vi "LCW_Flow_Mon_Main.vi"() -> ()   [LabVIEW 2019]
uses:
  <vilib>/MakerHub/LINX/LMH-LINX.lvlib
panel:
  in  "Logging":bool=TRUE
  out "Logging Status":bool
  in  "Tab Control":enum32{"Flow Chart", "Raw Voltage Chart"}(tab)
  out "M1 Chart":waveform(dbl)[](graph)
  out "M2 Chart":waveform(dbl)[](graph)
  out "M3 Chart":waveform(dbl)[](graph)
  out "M4 Chart":waveform(dbl)[](graph)
  out "WFS1 Chart":waveform(dbl)[](graph)
  out "M1 Voltage Chart":waveform(dbl)[](graph)
  out "M2 Voltage Chart":waveform(dbl)[](graph)
  out "M3 Voltage Chart":waveform(dbl)[](graph)
  out "M4 Voltage Chart":waveform(dbl)[](graph)
  out "WFS1 Voltage Chart":waveform(dbl)[](graph)
  out "M1_V":dbl caption="V" format="%.2g"
  out "M4_V":dbl caption="V" format="%.2g"
  out "M3_V":dbl caption="V" format="%.2g"
  out "M2_V":dbl caption="V" format="%.2g"
  out "WFS1_V":dbl caption="V" format="%.2g"
  out "Meas. steps":i32
  in  "n_avg":i32=1000 caption="N of samples per meas."
  out "WFS1":dbl format="%.2g"
  in  "VISA":refnum<visa-resource-name>="COM25"
  out "M4":dbl format="%.2g"
  out "M3":dbl format="%.2g"
  in  "Meas. Interval":i32=30
  out "M2":dbl format="%.2g"
  out "M1":dbl format="%.2g"
  out "Readout Status":bool
  out "Last Measured":timestamp format="%<%Y-%m-%d %H:%M:%S>T"
  in  "Stop":bool
  # "LCW Flow Monitor"
  # "sec"
  # "("
  # ")"
  # "GPM"
  # "GPM"
  # "GPM"
  # "GPM"
  # "GPM"
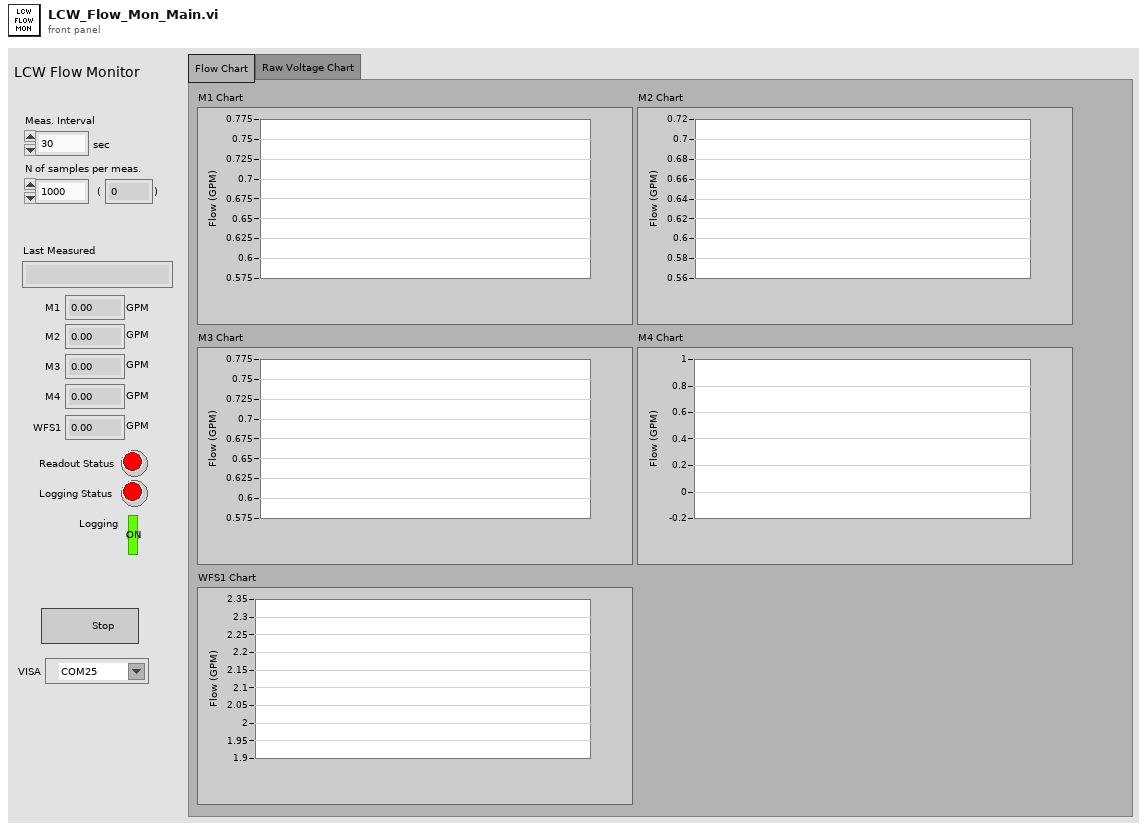
[diagram p1: front panel]
types:
  T1 = typedef "LMH-LINX.lvlib/LINX Ref.ctl" = cluster{"IO":T2, "Interface":T3, "LINX Device Config":T4}
  T2 = typedef "LMH-LINX.lvlib/Platform.ctl" = enum16{"Remote", "Local"}
  T3 = typedef "LMH-LINX.lvlib/Interface.ctl" = enum16{"Serial", "TCP"}
  T4 = typedef "LMH-LINX.lvlib/Device.lvlib/LINX Device Config.ctl" = cluster{"Interface":T3, "COM Port":refnum<visa-resource-name>, "TCP Configuration":T5, "Device Family":u8, "Device ID":u8, "Device Name":string, "TCP Ref":refnum<k5>, "Channels":T6}
  T5 = typedef "LMH-LINX.lvlib/Device.lvlib/TCP Config.ctl" = cluster{"IP Address":string, "Port":u16}
  T6 = typedef "LMH-LINX.lvlib/Channels.ctl" = cluster{"DI":u8[], "DO":u8[], "AI":u8[], "AO":u8[], "PWM":u8[], "QE":u8[], "UART":u8[], "I2C 2":u8[], "SPI":u8[], "CAN":u8[], "Servo":u8[], "AI Ref (V)":dbl, "AI Resolution (Bits)":u8, "AO Ref (V)":dbl, "AO Resolution (Bits)":u8}
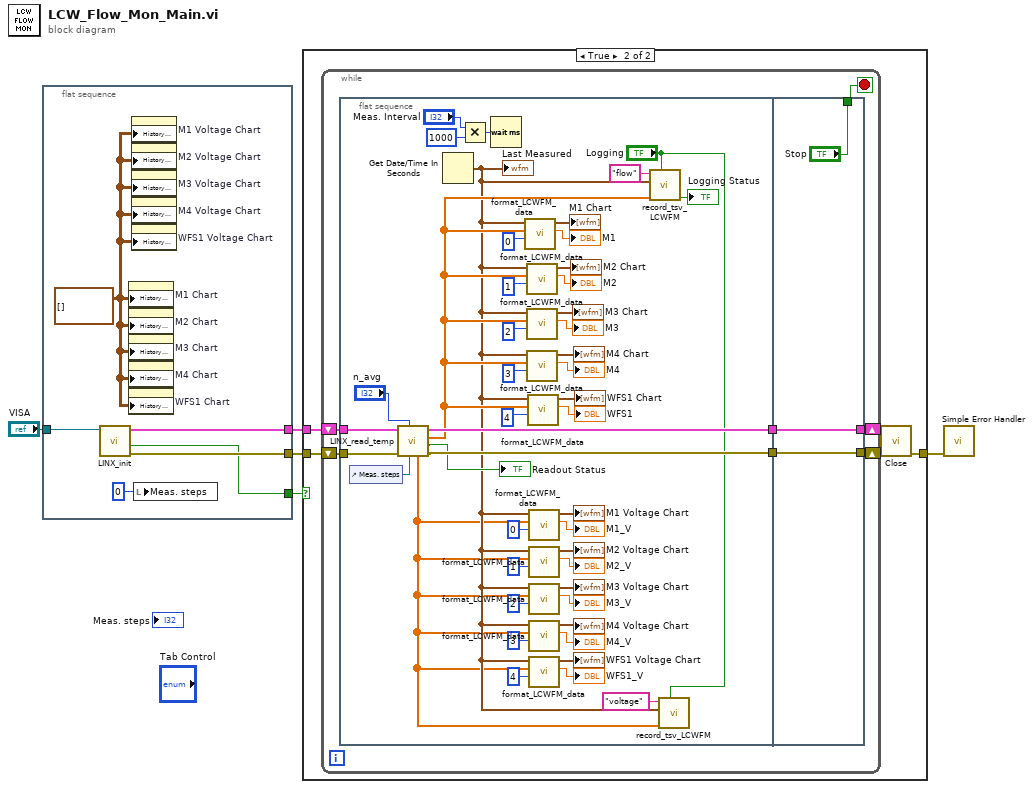
[diagram p0: block diagram]
diagram:
  n1 = flat-sequence {
    tunnel: [w8] -> w4
    tunnel: [w11] -> w3
    tunnel: "VISA" -> [w10]
    tunnel: [w9] -> w1
    frame #0 {
      w6 = waveform(dbl)[][] [] ("History Data")
      n2 = call "LINX_init.vi"("VISA"=w10) -> ("error out"=w11:errorcluster, "status"=w8:bool, "LINX Resource"=w9:T1)  [unwired: 8 in]
      n3 = property on="M1 Chart" class="WFChart (strict)"("History Data"=w6) -> ()  [unwired: 2 in, 2 out]
      n4 = property on="M2 Chart" class="WFChart (strict)"("History Data"=w6) -> ()  [unwired: 2 in, 2 out]
      n5 = property on="M3 Chart" class="WFChart (strict)"("History Data"=w6) -> ()  [unwired: 2 in, 2 out]
      n6 = property on="M4 Chart" class="WFChart (strict)"("History Data"=w6) -> ()  [unwired: 2 in, 2 out]
      n7 = property on="WFS1 Chart" class="WFChart (strict)"("History Data"=w6) -> ()  [unwired: 2 in, 2 out]
      n8 = property on="M1 Voltage Chart" class="WFChart (strict)"("History Data"=w6) -> ()  [unwired: 2 in, 2 out]
      n9 = property on="M2 Voltage Chart" class="WFChart (strict)"("History Data"=w6) -> ()  [unwired: 2 in, 2 out]
      n10 = property on="M3 Voltage Chart" class="WFChart (strict)"("History Data"=w6) -> ()  [unwired: 2 in, 2 out]
      n11 = property on="M4 Voltage Chart" class="WFChart (strict)"("History Data"=w6) -> ()  [unwired: 2 in, 2 out]
      n12 = property on="WFS1 Voltage Chart" class="WFChart (strict)"("History Data"=w6) -> ()  [unwired: 2 in, 2 out]
      n13 = local write "Meas. steps"(0 ("Meas. steps")) -> ()
    }
  }
  n14 = case shown="True" w4 {
    tunnel: [w12 w15] -> w5
    tunnel: w3 -> [w12 w17]
    tunnel: w1 -> [_ w16]
    frame False {
    }
    frame True {
      n15 = while {
        shift-right: [w21] -> w14
        shift-left: w17 -> [w24]
        shift-right: [w22] -> w13
        shift-left: w16 -> [w23]
        stop <- w18 stop-if-true
        n16 = flat-sequence {
          tunnel: w24 -> [w68]
          tunnel: w23 -> [w67]
          tunnel: [w66] -> w20
          tunnel: [w65] -> w19
          tunnel: [w73] -> w21
          tunnel: [w74] -> w22
          tunnel: w20 -> [w74]
          tunnel: w19 -> [w73]
          tunnel: ["Stop"] -> w18
          frame #0 {
            n17 = control-ref of="Meas. steps"() -> (w61:refnum<vi>)
            n18 = call "LINX_read_temp.vi"("n_step"=w61, "n_avg"="n_avg", "Error In"=w68, "LINX Resource"=w67) -> ("Error Out"=w65:errorcluster, "status"=→"Readout Status":bool, "array_flow"=w49:dbl[], "LINX Resource Out"=w66:T1, "array_voltage"=w31:dbl[])  [unwired: 3 in]
            n19 = Get Date/Time In Seconds() -> (seconds since 1Jan1904=w32:timestamp)
            "Last Measured" <- w32
            n20 = Multiply(x="Meas. Interval", y=1000) -> (x*y=w27:i32)
            n21 = Wait (ms)(milliseconds to wait=w27) -> ()  [unwired: 1 out]
            n22 = call "format_LCWFM_data.vi"("index"=0, "value_array"=w49, "time"=w32) -> ("value"=→"M1":dbl, "waveform_array"=→"M1 Chart":waveform(dbl)[])  [unwired: 7 in]
            n23 = call "format_LCWFM_data.vi"("index"=1, "value_array"=w49, "time"=w32) -> ("value"=→"M2":dbl, "waveform_array"=→"M2 Chart":waveform(dbl)[])  [unwired: 7 in]
            n24 = call "format_LCWFM_data.vi"("index"=2, "value_array"=w49, "time"=w32) -> ("value"=→"M3":dbl, "waveform_array"=→"M3 Chart":waveform(dbl)[])  [unwired: 7 in]
            n25 = call "format_LCWFM_data.vi"("index"=3, "value_array"=w49, "time"=w32) -> ("value"=→"M4":dbl, "waveform_array"=→"M4 Chart":waveform(dbl)[])  [unwired: 7 in]
            n26 = call "format_LCWFM_data.vi"("index"=4, "value_array"=w49, "time"=w32) -> ("value"=→"WFS1":dbl, "waveform_array"=→"WFS1 Chart":waveform(dbl)[])  [unwired: 7 in]
            n27 = call "format_LCWFM_data.vi"("index"=0, "value_array"=w31, "time"=w32) -> ("value"=→"M1_V":dbl, "waveform_array"=→"M1 Voltage Chart":waveform(dbl)[])  [unwired: 7 in]
            n28 = call "format_LCWFM_data.vi"("index"=1, "value_array"=w31, "time"=w32) -> ("value"=→"M2_V":dbl, "waveform_array"=→"M2 Voltage Chart":waveform(dbl)[])  [unwired: 7 in]
            n29 = call "format_LCWFM_data.vi"("index"=2, "value_array"=w31, "time"=w32) -> ("value"=→"M3_V":dbl, "waveform_array"=→"M3 Voltage Chart":waveform(dbl)[])  [unwired: 7 in]
            n30 = call "format_LCWFM_data.vi"("index"=3, "value_array"=w31, "time"=w32) -> ("value"=→"M4_V":dbl, "waveform_array"=→"M4 Voltage Chart":waveform(dbl)[])  [unwired: 7 in]
            n31 = call "format_LCWFM_data.vi"("index"=4, "value_array"=w31, "time"=w32) -> ("value"=→"WFS1_V":dbl, "waveform_array"=→"WFS1 Voltage Chart":waveform(dbl)[])  [unwired: 7 in]
            n32 = call "record_tsv_LCWFM.vi"("record_on"="Logging", "value_array"=w49, "time"=w32, "file_name"="flow") -> ("status"=→"Logging Status":bool)  [unwired: 7 in]
            n33 = call "record_tsv_LCWFM.vi"("record_on"="Logging", "value_array"=w31, "time"=w32, "file_name"="voltage") -> ()  [unwired: 7 in, 1 out]
          }
          frame #1 {
          }
        }
      }
      n34 = call <vilib>:"Close.vi"("Error In"=w14, "LINX Resource"=w13) -> ("Error Out"=w15:errorcluster)  [unwired: 9 in]
    }
  }
  n35 = call <vilib>:"Simple Error Handler.vi"("error in (no error)"=w5) -> ()  [unwired: 4 in, 5 out]
